vi "FlipMirror.vi"() -> ()   [LabVIEW 2009]
uses:
  <vilib>/DAQmx/write.llb/DAQmx Write (Digital Bool 1Line 1Point).vi
panel:
  in  "Galvo Pos":dbl
  in  "AOD Pos":dbl=25.0
  in  "HWSerialNum":i32=83823342
  in  "MG17Motor":refnum<k7>(container)
  in  "AOD":bool
  in  "Stop":bool
  in  "Flip":bool
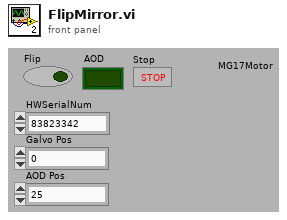
[diagram p1: front panel]
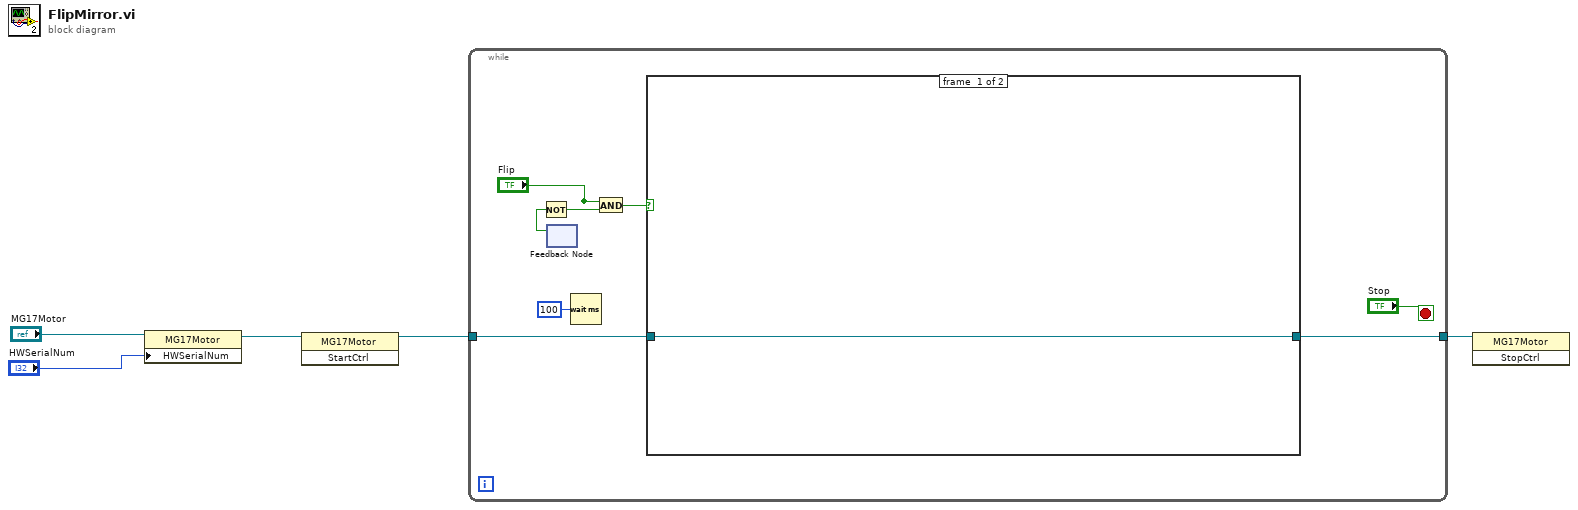
[diagram p0: block diagram]
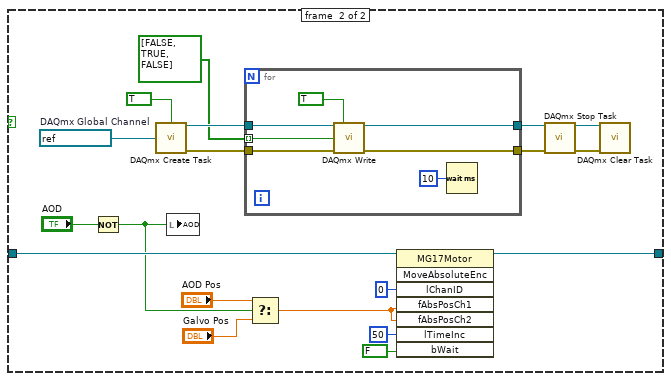
[diagram p2: hidden frame]
diagram:
  n1 = property class="MG17Motor"(reference="MG17Motor", "HWSerialNum"="HWSerialNum") -> (reference out=w3:refnum<k7>)  [unwired: 1 in, 1 out]
  n2 = invoke class="MG17Motor" method="StartCtrl"(reference=w3) -> (reference out=w2:refnum<k7>)  [unwired: 2 in, 2 out]
  n3 = while {
    tunnel: w2 -> [w7]
    tunnel: [w6] -> w1
    stop <- "Stop" stop-if-true
    n4 = feedback #1() -> (w13:bool)  [unwired: 1 in]
    n5 = Not(x=w13) -> (.not. x?=w12:bool)
    n6 = Wait (ms)(milliseconds to wait=u32 100) -> ()  [unwired: 1 out]
    n7 = And(x="Flip", y=w12) -> (x .and. y?=w10:bool)
    n8 = case shown="True" w10 {
      tunnel: w7 -> [w14 w23]
      tunnel: [w14 w22] -> w6
      frame #0 {
      }
      frame #1 {
        w28 = refnum<k21> "FlipMirror"  # DAQmx Global Channel
        n9 = Not(x="AOD") -> (.not. x?=w18:bool)
        n10 = call <vilib>:"DAQmx Create Task.vi"("auto cleanup"=TRUE, "global virtual channels"=w28) -> ("task out"=w27:refnum<k21>, "error out"=w26:errorcluster)  [unwired: 12 in]
        n11 = local write "AOD"(w18) -> ()
        n12 = for {
          tunnel: [w40] -> w32
          tunnel: [w39] -> w31
          tunnel: w27 -> [w37]
          tunnel: w26 -> [w36]
          tunnel: bool[] [FALSE, TRUE, FALSE] -> [w35] mode=indexing
          n13 = call-poly <vilib>:"DAQmx Write.vi"("task/channels in"=w37, "auto start"=TRUE, "data"=w35, "error in"=w36) -> ("task out"=w40:refnum<k21>, "error out"=w39:errorcluster)  [unwired: 9 in, 1 out]
          n14 = Wait (ms)(milliseconds to wait=u32 10) -> ()  [unwired: 1 out]
        }
        n15 = Select(t="AOD Pos", s=w18, f="Galvo Pos") -> (s? t:f=w15:dbl)
        n16 = invoke class="MG17Motor" method="MoveAbsoluteEnc"(reference=w23, "lChanID"=0, "fAbsPosCh1"=w15, "fAbsPosCh2"=w15, "lTimeInc"=50, "bWait"=FALSE) -> (reference out=w22:refnum<k7>)  [unwired: 2 in, 7 out]
        n17 = call <vilib>:"DAQmx Stop Task.vi"("task/channels in"=w32, "error in"=w31) -> ("task out"=w30:refnum<k21>, "error out"=w29:errorcluster)  [unwired: 12 in]
        n18 = call <vilib>:"DAQmx Clear Task.vi"("task in"=w30, "error in"=w29) -> ()  [unwired: 13 in, 1 out]
      }
    }
  }
  n19 = invoke class="MG17Motor" method="StopCtrl"(reference=w1) -> ()  [unwired: 2 in, 3 out]
